vi "lab_1.2.vi"() -> ()   [LabVIEW 2022 SP3]
panel:
  out "Z":dbl
  in  "Y":dbl
  in  "X":dbl
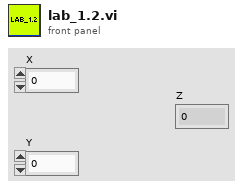
[diagram p1: front panel]
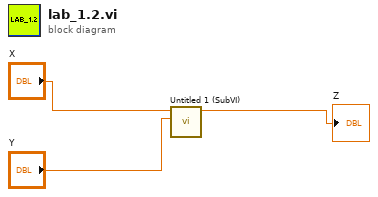
[diagram p0: block diagram]
diagram:
  n1 = call "Untitled 1 (SubVI).vi"("Y"="Y", "X"="X") -> ("z"=→"Z":dbl)  [unwired: 9 in]
